vi "CANTest.vi"() -> ()   [LabVIEW 2009]
uses:
  SubVIs/CAN Jaguar Control Mode.ctl
  SubVIs/CAN Jaguar Position Reference.ctl
  <vilib>/Platform/TimedLoop/XDataNode/XDataNode.xnode
  <vilib>/Platform/TimedLoop/XDataNode/loadlvalarms.vi
  <vilib>/Platform/TimedLoop/XDataNode/timing_clust.ctl
  <vilib>/Platform/TimedLoop/XDataNode/nitl_modes.ctl
  <vilib>/Platform/TimedLoop/XDataNode/wakeup.ctl
  Serial.lvlib
  <vilib>/Platform/TimedLoop/XDataNode/XDNodeRunTimeDep.lvlib
  CAN.lvlib
panel:
  in  "Encoder Initial Position":dbl
  in  "Output Set Point":dbl
  out "D 2":dbl
  out "I 2":dbl
  out "P 2":dbl
  out "Output Set Point 2":dbl
  in  "Maximum Output Voltage":dbl=4.0
  in  "D":dbl
  in  "I":dbl=0.1
  in  "P":dbl=100.0
  in  "Device Number":u8=2
  out "error out 2":errorcluster
  out "error out":errorcluster
  in  "stop":bool
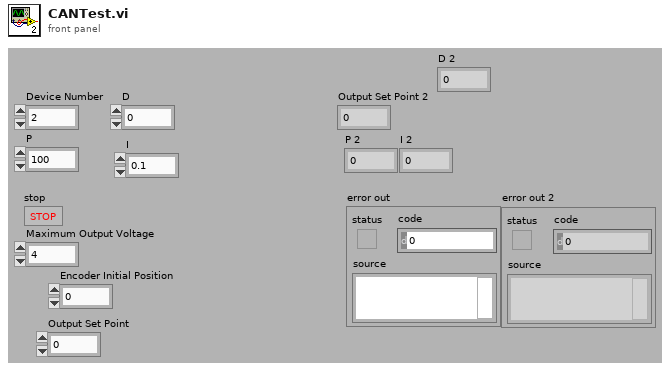
[diagram p1: front panel]
types:
  T1 = typedef "CAN.lvlib/CAN Jaguar Position Reference.ctl" = enum16{"Encoder", "Potentiometer"}
  T2 = typedef "CAN.lvlib/CAN Jaguar Control Mode.ctl" = enum16{"Percent VBus", "Speed", "Position", "Current"}
  T3 = typedef "XDNodeRunTimeDep.lvlib/timing_clust.ctl" = cluster{"Expected End [f-1]":u64, "Actual End [f-1]":u64, "Finished Late? [f-1]":bool, "Expected End [i-1]":u64, "Actual End [i-1]":u64, "Finished Late? [i-1]":bool, "Expected Start [i]":u64, "Actual Start [i]":u64, "Expected Start [f]":u64, "Actual Start [f]":u64, "Source Name":string, "Structure Name":string, "Period":i64, "Deadline":i64, "Offset":i64, "Start":i64, "Priority":i32, "Timeout":i32, "Mode":T4, "Wakeup Reason":T5, "Error":errorcluster, "Source Type":string, "Secondary Source Type":string, "Global End Time":u64, "Global Start Time":u64, "Frame Duration":u64, "Iteration Duration":u64, "Assigned CPU":i32, "I/O Scan Engine Mode":u32}
  T4 = typedef "XDNodeRunTimeDep.lvlib/nitl_modes.ctl" = enum32{"No Change", "Process missed periods, maintain original phase", "Discard missed periods, maintain original phase", "Process missed periods, ignore original phase", "Discard missed periods, ignore original phase"}
  T5 = typedef "XDNodeRunTimeDep.lvlib/wakeup.ctl" = enum32{"Normal", "Aborted", "Asynchronous wakeup", "Timing source error", "Timed loop error", "Timeout"}
  T6 = typedef "CAN.lvlib/CAN Jaguar Ref.ctl" = cluster{"Device Number":u8, "Control Mode":T2, "Inverted":bool, "Semaphore":T7, "Max Vout":dbl, "DevStatus":errorcluster}
  T7 = typedef "Semaphore RefNum" = refnum<k1>
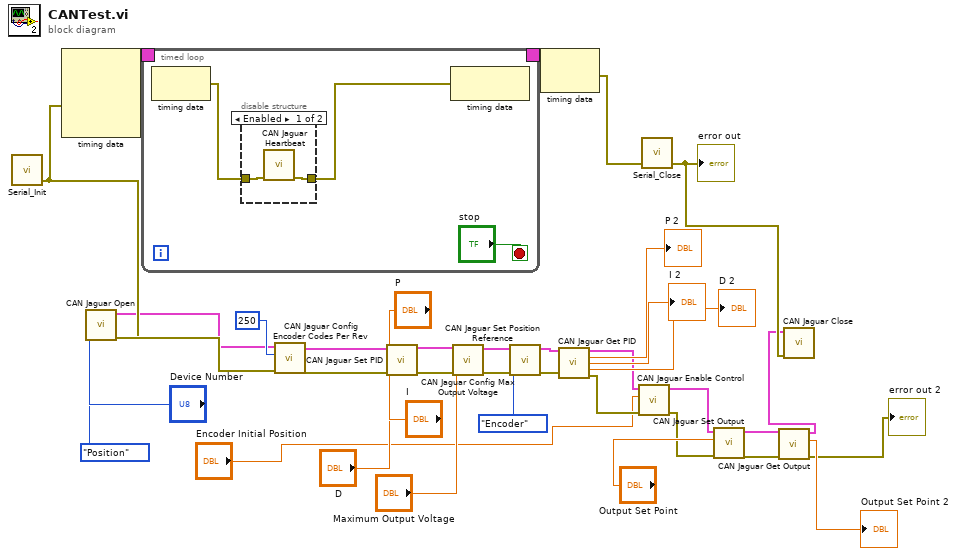
[diagram p0: block diagram]
diagram:
  n1 = call "Serial_Init.vi"() -> ("error out"=w16:errorcluster)  [unwired: 4 in, 1 out]
  n2 = node-c288(w16) -> (w37:T3)  [unwired: 3 in]
  n3 = call "CAN Jaguar Open.vi"("error in (no error)"=w16, "Control Mode"=CAN_Jaguar_Control_Mode."Position", "Device Number"="Device Number") -> ("error out"=w32:errorcluster, "CAN Jaguar Ref Out"=w15:T6)  [unwired: 7 in]
  n4 = timed-loop {
    timing: w37 -> [_]
    timing-out: [_] -> w36
    stop <- "stop" stop-if-true
    n5 = node-c288() -> (w40:errorcluster)  [unwired: 1 in]
    n6 = disable-structure shown="Enabled" {
      disable-tunnel: w40 -> [w42 _]
      disable-tunnel: [w41 _] -> w39
      frame #0 {
        n7 = call "CAN Jaguar Heartbeat.vi"("error in (no error)"=w42) -> ("error out"=w41:errorcluster)  [unwired: 10 in]
      }
      frame #1 {
      }
    }
    n8 = node-c288(w39) -> ()  [unwired: 1 out]
  }
  n9 = call "CAN Jaguar Config Encoder Codes Per Rev.vi"("error in (no error)"=w32, "Encoder Codes Per Rev"=u16 250, "CAN Jaguar Ref"=w15) -> ("error out"=w6:errorcluster, "CAN Jaguar Ref Out"=w7:T6)  [unwired: 7 in]
  n10 = call "CAN Jaguar Set PID.vi"("CAN Jaguar Ref"=w7, "P"="P", "I"="I", "D"="D", "error in (no error)"=w6) -> ("CAN Jaguar Ref Out"=w27:T6, "error out"=w26:errorcluster)  [unwired: 9 in]
  n11 = call "CAN Jaguar Config Max Output Voltage.vi"("error in (no error)"=w26, "Maximum Output Voltage"="Maximum Output Voltage", "CAN Jaguar Ref"=w27) -> ("error out"=w23:errorcluster, "CAN Jaguar Ref Out"=w24:T6)  [unwired: 7 in]
  n12 = call "CAN Jaguar Set Position Reference.vi"("error in (no error)"=w23, "Position Reference"=CAN_Jaguar_Position_Reference."Encoder", "CAN Jaguar Ref"=w24) -> ("error out"=w20:errorcluster, "CAN Jaguar Ref Out"=w21:T6)  [unwired: 7 in]
  n13 = node-c288(w36) -> (w35:errorcluster)
  n14 = call "CAN Jaguar Get PID.vi"("CAN Jaguar Ref"=w21, "error in (no error)"=w20) -> ("CAN Jaguar Ref Out"=w5:T6, "P"=→"P 2":dbl, "I"=→"I 2":dbl, "D"=→"D 2":dbl, "error out"=w4:errorcluster)  [unwired: 9 in]
  n15 = call "CAN Jaguar Enable Control.vi"("error in (no error)"=w4, "Encoder Initial Position"="Encoder Initial Position", "CAN Jaguar Ref"=w5) -> ("error out"=w3:errorcluster, "CAN Jaguar Ref Out"=w2:T6)  [unwired: 7 in]
  n16 = call "Serial_Close.vi"("error in (no error)"=w35) -> ("error out"=w14:errorcluster)  [unwired: 4 in]
  "error out" <- w14
  n17 = call "CAN Jaguar Set Output.vi"("error in (no error)"=w3, "Output Set Point"="Output Set Point", "CAN Jaguar Ref"=w2) -> ("error out"=w12:errorcluster, "CAN Jaguar Ref Out"=w11:T6)  [unwired: 7 in]
  n18 = call "CAN Jaguar Get Output.vi"("error in (no error)"=w12, "CAN Jaguar Ref"=w11) -> ("error out"=→"error out 2":errorcluster, "Output Set Point"=→"Output Set Point 2":dbl, "CAN Jaguar Ref Out"=w9:T6)  [unwired: 7 in]
  n19 = call "CAN Jaguar Close.vi"("error in (no error)"=w14, "CAN Jaguar Ref"=w9) -> ()  [unwired: 9 in, 1 out]
